vi "Decide Image decimation.vi"(5 "FPS":dbl, 9 "Max bytes per sec":u32=100000000, 10 "Image decimation counter in":u32, 11 "element in":T2) -> (1 "Image decimation counter out":u32, 2 "send current image data":bool)   [LabVIEW 2025, in "Automotive Vision.lvclass"]
doc: "Decide to skip the current frame based on settings (what is the maximum bytes per second to transfer) and image data (resolution, image type, FPS)."
uses:
  Automotive Vision.lvclass
  <instrlib>/FlexRIO/CSI-2/v2/Common/Types/LLP Data Type.ctl
  Automotive Vision.lvclass/Automotive Vision.ctl
  <instrlib>/FlexRIO/CSI-2/v2/Common/NI CSI-2 API Common v2.lvlib
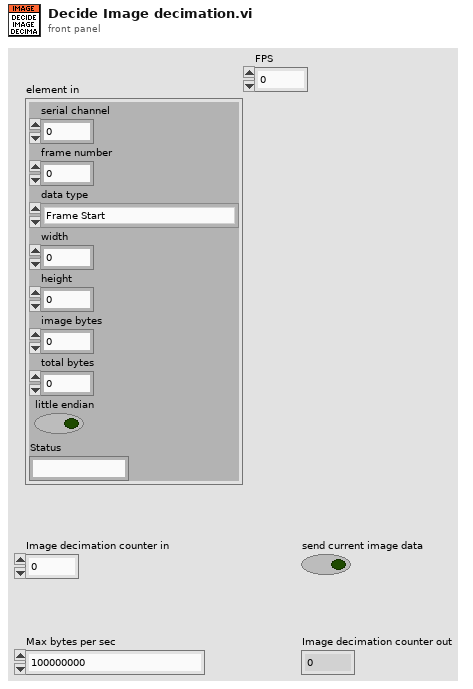
[diagram p1: front panel]
types:
  T1 = typedef "NI CSI-2 API Common v2.lvlib/LLP Data Type.ctl" = enum8{"Frame Start", "Frame End", "Line Start", "Line End", "End of Transmission", "Reserved 0", "Reserved 1", "Reserved 2", "Generic Short Packet 1", "Generic Short Packet 2", "Generic Short Packet 3", "Generic Short Packet 4", "Generic Short Packet 5", "Generic Short Packet 6", "Generic Short Packet 7", "Generic Short Packet 8", "Null", "Blanking Data", "Embedded 8-bit non Image Data", "Generic Long Packet 1", "Generic Long Packet 2", "Generic Long Packet 3", "Generic Long Packet 4", "Reserved 3", "YUV420 8-bit", "YUV420 10-bit", "Legacy YUV420 8-bit", "Reserved 4", "YUV420 8-bit Chroma Shifted", "YUV420 10-bit Chroma Shifted", "YUV422 8-bit", "YUV422 10-bit", "RGB444", "RGB555", "RGB565", "RGB666", "RGB888", "Reserved 5", "Reserved 6", "RAW 24", "RAW 6", "RAW 7", "RAW 8", "RAW 10", "RAW 12", "RAW 14", "RAW 16", "RAW 20", "User Defined 8-bit Data 1", "User Defined 8-bit Data 2", "User Defined 8-bit Data 3", "User Defined 8-bit Data 4", "User Defined 8-bit Data 5", "User Defined 8-bit Data 6", "User Defined 8-bit Data 7", "User Defined 8-bit Data 8", "USL Command", "Reserved 7", "Reserved 8", "Reserved 9", "Reserved 10", "Reserved 11", "Reserved 12", "LRTE EPD Spacer"}
  T2 = cluster{"serial channel":fxp<+,3,3>, "frame number":u16, "data type":T1, "width":u16, "height":u16, "image bytes":u32, "total bytes":u32, "little endian":bool, "Status":string}
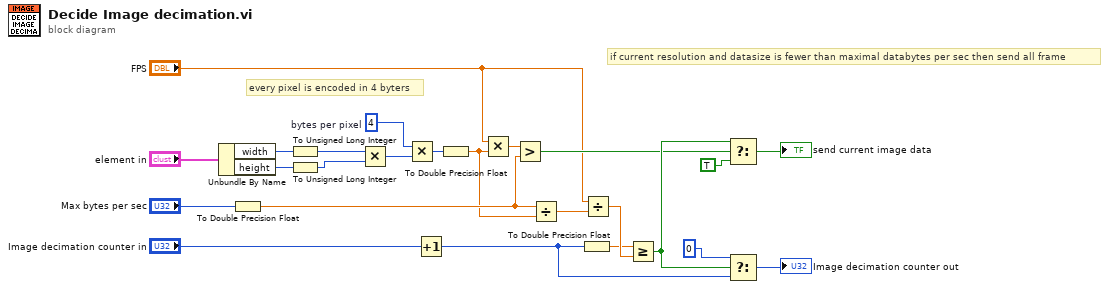
[diagram p0: block diagram]
diagram:
  w17 = u32 4  # bytes per pixel
  # "every pixel is encoded in 4 byters"
  # "if current resolution and datasize is fewer than maximal databytes per sec then send all frame"
  n1 = Unbundle By Name("element in") -> ("width"=w13:u16, "height"=w12:u16)
  n2 = To Double Precision Float(number="Max bytes per sec") -> (double precision float=w5:dbl)
  n3 = To Unsigned Long Integer(number=w13) -> (unsigned 32bit integer=w11:u32)
  n4 = To Unsigned Long Integer(number=w12) -> (unsigned 32bit integer=w10:u32)
  n5 = Multiply(x=w11, y=w10) -> (x*y=w18:u32)
  n6 = Multiply(x=w17, y=w18) -> (x*y=w4:u32)
  n7 = Increment(x="Image decimation counter in") -> (x+1=w2:u32)
  n8 = To Double Precision Float(number=w4) -> (double precision float=w3:dbl)
  n9 = Multiply(x="FPS", y=w3) -> (x*y=w9:dbl)
  n10 = Greater?(x=w9, y=w5) -> (0:w16:bool)
  n11 = Divide(x=w5, y=w3) -> (x/y=w14:dbl)
  n12 = To Double Precision Float(number=w2) -> (double precision float=w1:dbl)
  n13 = Divide(x="FPS", y=w14) -> (x/y=w15:dbl)
  n14 = Greater Or Equal?(x=w1, y=w15) -> (x >= y?=w22:bool)
  n15 = Select(t=w22, s=w16, f=TRUE) -> (s? t:f=→"send current image data":bool)
  n16 = Select(t=u32 0 ("y"), s=w22, f=w2) -> (s? t:f=→"Image decimation counter out":u32)
